vi "Stevci_Globals.vi"() -> ()   [LabVIEW 2021]
panel:
  in  "zacetni cas":dbl
  in  "casovna razlika":dbl
  in  "Števec vseh skokov 6":dbl
  in  "Števec skokov 6":dbl
  in  "Števec vseh skokov 5":dbl
  in  "Števec skokov 5":dbl
  in  "Števec vseh skokov 4":dbl
  in  "Števec skokov 4":dbl
  in  "Števec vseh skokov 3":dbl
  in  "Števec skokov 3":dbl
  in  "Števec vseh skokov 2":dbl
  in  "Števec skokov 2":dbl
  in  "Števec vseh skokov":dbl
  in  "Števec skokov":dbl
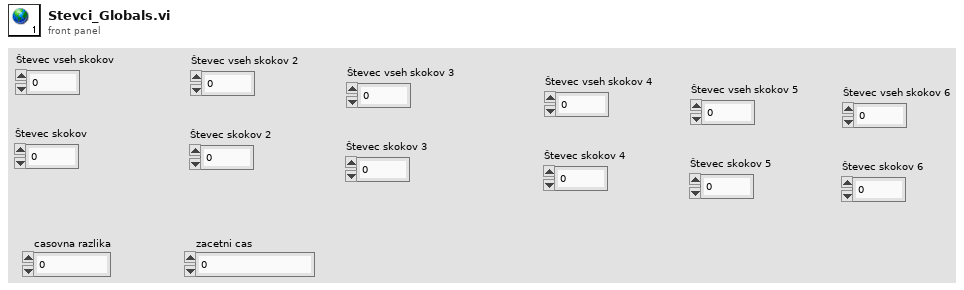
[diagram p1: front panel]
diagram:
